vi "DSF.Engine.Hardware Info.Create.vi"(8 "error in (no error)":errorcluster) -> (0 "error out":errorcluster, 3 "Hardware Info":refnum<class "DSF.Engine.Hardware Info.lvclass">)   [LabVIEW 2017, in "DSF.Engine.lvlib" / "DSF.Engine.Hardware Info.lvclass"]
uses:
  DSF.Engine.Hardware Info.lvclass
  DSF.Engine.Hardware Info.lvclass/DSF.Engine.Hardware Info.ctl
  DSF.Engine.Hardware Info.CPU.lvclass
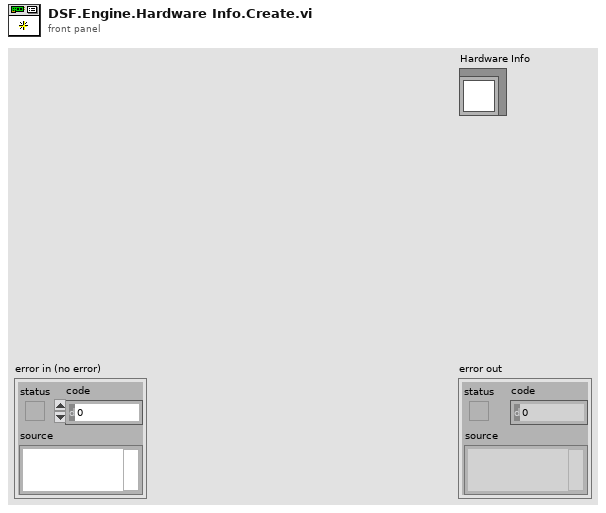
[diagram p1: front panel]
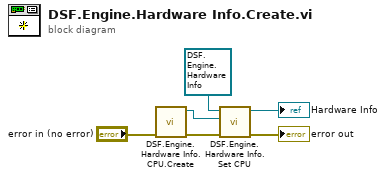
[diagram p0: block diagram]
diagram:
  n1 = call "DSF.Engine.Hardware Info.CPU.Create.vi"("error in (no error)"="error in (no error)") -> ("error out"=w1:errorcluster, "CPU Info out"=w5:refnum<class "DSF.Engine.Hardware Info.CPU.lvclass">)  [unwired: 9 in]
  n2 = call "DSF.Engine.Hardware Info.Set CPU.vi"("error in (no error)"=w1, "CPU Info"=w5, "Hardware Info in"=refnum<class "DSF.Engine.Hardware Info.lvclass"> refnum) -> ("error out"=→"error out":errorcluster, "Hardware Info out"=→"Hardware Info":refnum<class "DSF.Engine.Hardware Info.lvclass">)  [unwired: 7 in]
